vi "Information.vi"(8 "error in (no error)":errorcluster, 9 "Context":T1, 10 "Information.lvclass":refnum<class "Information.lvclass">, 11 "Publisher Actor in":refnum<class "Publisher Actor.lvclass">) -> (0 "error out":errorcluster, 3 "Publisher Actor out":refnum<class "Publisher Actor.lvclass">)   [LabVIEW 2021, in "Publisher Actor.lvclass"]
uses:
  Publisher Actor.lvclass
  Interfaces/Information/Information.lvclass
  Context.ctl
  Publisher Actor.lvclass/Publisher Actor.ctl
  Interfaces/Subscriber Messages/Information Msg/Information Msg.lvclass/Information Msg.ctl
  <vilib>/ActorFramework/Message Enqueuer/Message Enqueuer.lvclass/Message Enqueuer.ctl
  8f954a23-01b0-4d42-b608-54ddebbb3dff.vi
  <vilib>/ActorFramework/Message Enqueuer/Enqueue.vi
  Interfaces/Subscriber Messages/Information Msg/Information Msg.lvclass
  C:/Program Files/National Instruments/LabVIEW 2021/vi.lib/ActorFramework/Message/Message.lvclass
  <vilib>/ActorFramework/Message Priority Queue/Priority Enqueue.vi
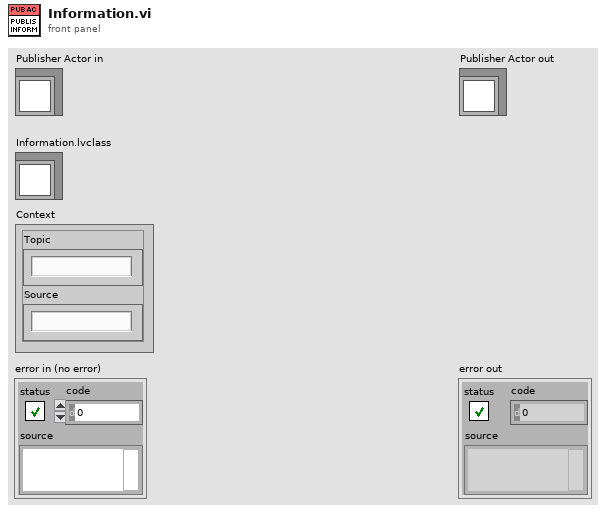
[diagram p1: front panel]
types:
  T1 = typedef "Context.ctl" = cluster{"Topic":string, "Source":string}
  T2 = map{T1, set{refnum<class "Message Enqueuer.lvclass">}}
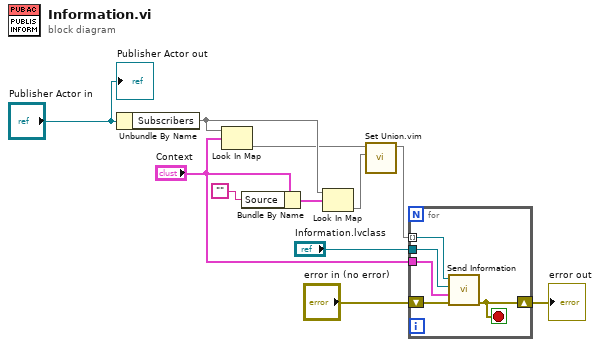
[diagram p0: block diagram]
diagram:
  n1 = Unbundle By Name("Publisher Actor in") -> ("Subscribers"=w6:T2)
  n2 = Look In Map(map=w6, key="Context") -> (value=w5:set{refnum<class "Message Enqueuer.lvclass">})  [unwired: 1 in, 1 out]
  n3 = Bundle By Name(cluster="Context", "Source"="") -> (w7:T1)
  n4 = Look In Map(map=w6, key=w7) -> (value=w4:set{refnum<class "Message Enqueuer.lvclass">})  [unwired: 1 in, 1 out]
  n5 = call "Set Union.vim"("set 2"=w4, "set 1"=w5) -> ("union"=w3:set{refnum<class "Message Enqueuer.lvclass">})  [unwired: 9 in]
  n6 = for {
    tunnel: w3 -> [w16] mode=indexing
    tunnel: "Information.lvclass" -> [w15]
    tunnel: "Context" -> [w14]
    shift-right: [w12] -> w1
    shift-left: "error in (no error)" -> [w13]
    stop <- w12 stop-if-true
    n7 = call "Send Information.vi"("error in (no error)"=w13, "Context"=w14, "Information"=w15, "Message Enqueuer"=w16) -> ("error out"=w12:errorcluster)  [unwired: 6 in, 1 out]
  }
  "error out" <- w1
  "Publisher Actor out" <- "Publisher Actor in"
